vi "AgilientVSGCtrl.vi"(7 "action":T1, 8 "error in (no error)":errorcluster, 10 "pow write":dbl, 11 "VISA resource name":refnum<visa-resource-name>="TCPIP0::192.168.1.203::inst0::INSTR") -> (0 "error out":errorcluster, 2 "pow read":dbl)   [LabVIEW 2019]
uses:
  controls/AgilentCtrlEnum.ctl
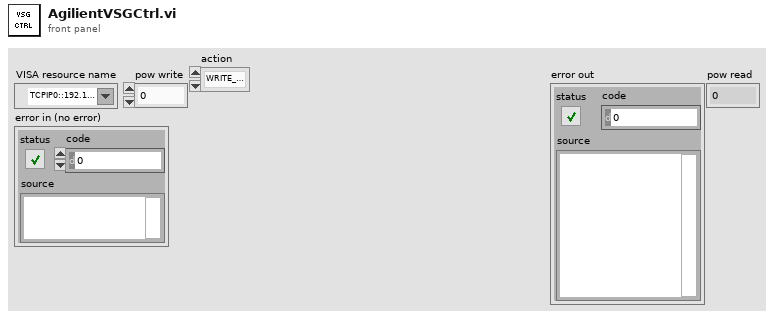
[diagram p1: front panel]
types:
  T1 = typedef "AgilentCtrlEnum.ctl" = enum16{"WRITE_POW", "READ_POW"}
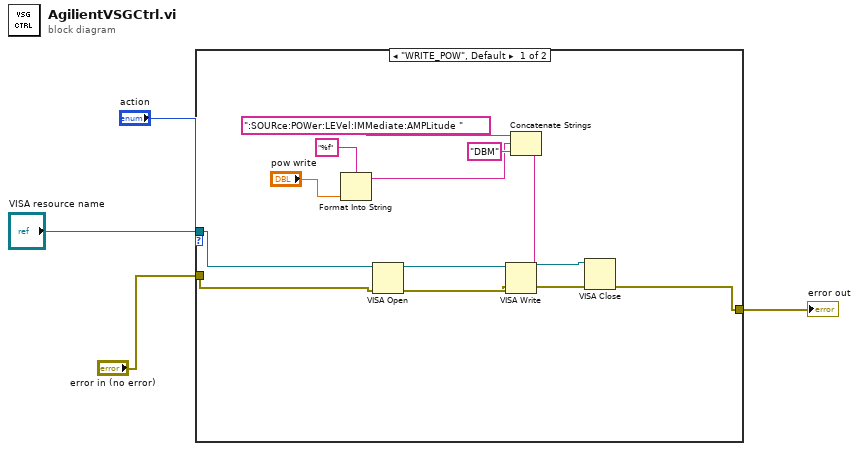
[diagram p0: block diagram]
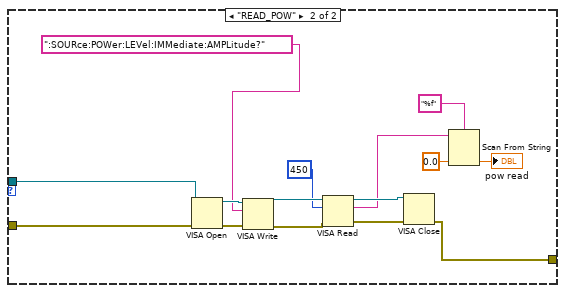
[diagram p2: hidden frame]
diagram:
  n1 = case shown="\"WRITE_POW\", Default" "action" {
    tunnel: "VISA resource name" -> [w10 w26]
    tunnel: "error in (no error)" -> [w9 w23]
    tunnel: [w6 w22] -> w2
    frame "WRITE_POW", Default {
      n2 = Format Into String(format string="%f", "pow write") -> (resulting string=w13:string)  [unwired: 2 in, 1 out]
      n3 = VISA Open(error in (no error)=w9, VISA resource name=w10) -> (VISA resource name=w11:refnum<visa-resource-name>, error out=w12:errorcluster)  [unwired: 3 in]
      n4 = Concatenate Strings(":SOURce:POWer:LEVel:IMMediate:AMPLitude " ("write buffer"), w13, "DBM" ("string")) -> (w5:string)
      n5 = VISA Write(VISA resource name=w11, write buffer=w5, error in (no error)=w12) -> (VISA resource name out=w8:refnum<visa-resource-name>, error out=w7:errorcluster)  [unwired: 1 out]
      n6 = VISA Close(VISA resource name=w8, error in (no error)=w7) -> (error out=w6:errorcluster)
    }
    frame "READ_POW" {
      n7 = VISA Open(error in (no error)=w23, VISA resource name=w26) -> (VISA resource name=w28:refnum<visa-resource-name>, error out=w29:errorcluster)  [unwired: 3 in]
      n8 = VISA Write(VISA resource name=w28, write buffer=":SOURce:POWer:LEVel:IMMediate:AMPLitude?", error in (no error)=w29) -> (VISA resource name out=w32:refnum<visa-resource-name>, error out=w31:errorcluster)  [unwired: 1 out]
      n9 = VISA Read(VISA resource name=w32, byte count=u32 450, error in (no error)=w31) -> (VISA resource name out=w25:refnum<visa-resource-name>, read buffer=w21:string, error out=w24:errorcluster)  [unwired: 1 out]
      n10 = VISA Close(VISA resource name=w25, error in (no error)=w24) -> (error out=w22:errorcluster)
      n11 = Scan From String(format string="%f", input string=w21, default 1=0.0 ("default value 1")) -> (output 1=→"pow read":dbl)  [unwired: 2 in, 3 out]
    }
  }
  "error out" <- w2
